vi "Table, Set Cell Value, Double.vi"(4 "format (%f)":string="%f", 5 "value":dbl format="%.6f", 6 "error in":errorcluster, 7 "column (0)":i32, 8 "row (0)":i32, 9 "Tbl Refnum":refnum<vi>) -> (0 "error out":errorcluster, 1 "column+1":i32, 2 "row+1":i32, 3 "Tbl Refnum out":refnum<vi>)   [LabVIEW 2010]
doc: "This function sets a single table cell double precision floating point value."
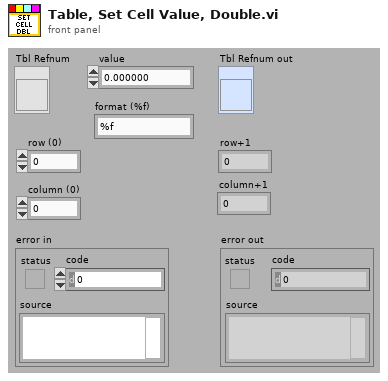
[diagram p1: front panel]
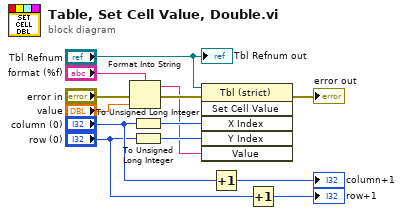
[diagram p0: block diagram]
diagram:
  n1 = Format Into String(format string="format (%f)", error in="error in", "value") -> (resulting string=w1:string, error out=w4:errorcluster)  [unwired: 1 in]
  n2 = To Unsigned Long Integer(number="column (0)") -> (unsigned 32bit integer=w7:u32)
  n3 = To Unsigned Long Integer(number="row (0)") -> (unsigned 32bit integer=w6:u32)
  n4 = invoke class="Tbl (strict)" method="Set Cell Value"(reference="Tbl Refnum", error in=w4, "X Index"=w7, "Y Index"=w6, "Value"=w1) -> (error out=→"error out":errorcluster)  [unwired: 1 in, 5 out]
  n5 = Increment(x="column (0)") -> (x+1=→"column+1":i32)
  n6 = Increment(x="row (0)") -> (x+1=→"row+1":i32)
  "Tbl Refnum out" <- "Tbl Refnum"
